vi "三转换ROI对比2.vi"() -> ()   [LabVIEW 2018]
uses:
  <vilib>/vision/NI_Vision_Development_Module.lvlib
panel:
  out "Image 4":T1(plugin-control)
  out "Image 3":T1(plugin-control)
  out "Image 2":T1(plugin-control)
  out "error out":errorcluster
  out "元素":T2 {"Contours"."Type" items=["No Selection", "Point", "Line", "Rectangle", "Oval", "Polygon", "Freehand Region", "Annulus", "Unused2", "Unused3", "Broken Line", "Freehand Line", "Rotated Rectangle"]}
  in  "索引":i32
  out "Image":T1(plugin-control)
  in  "路径":path
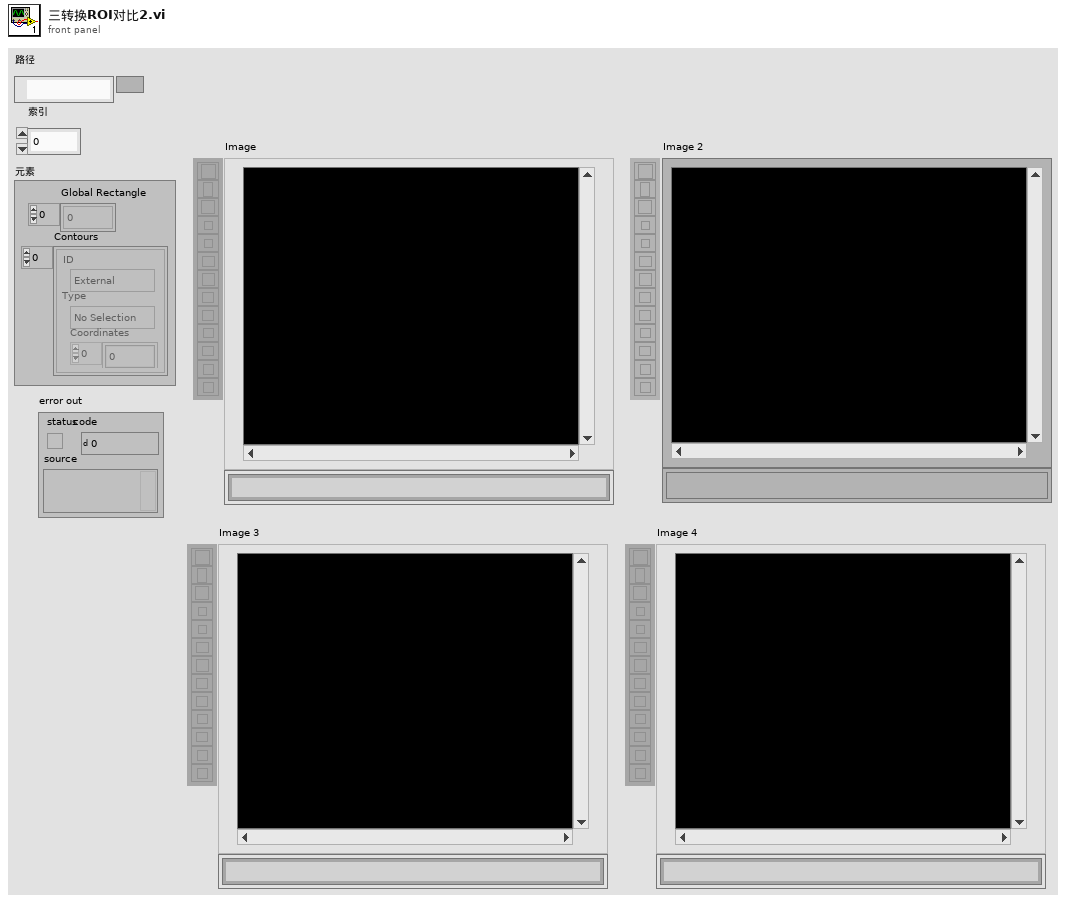
[diagram p1: front panel]
types:
  T1 = typedef "IMAQ Image.ctl" = refnum<image>
  T2 = typedef "ROI Descriptor" = cluster{"Global Rectangle":i32[], "Contours":cluster{"ID":enum32{"External", "Internal"}, "Type":u32, "Coordinates":i32[]}[]}
  T3 = typedef "Image Type" = u32
  T4 = cluster{"ID":enum32{"External", "Internal"}, "Type":u32, "Coordinates":i32[]}[]
  T5 = cluster{"ID":enum32{"External", "Internal"}, "Type":u32, "Coordinates":i32[]}
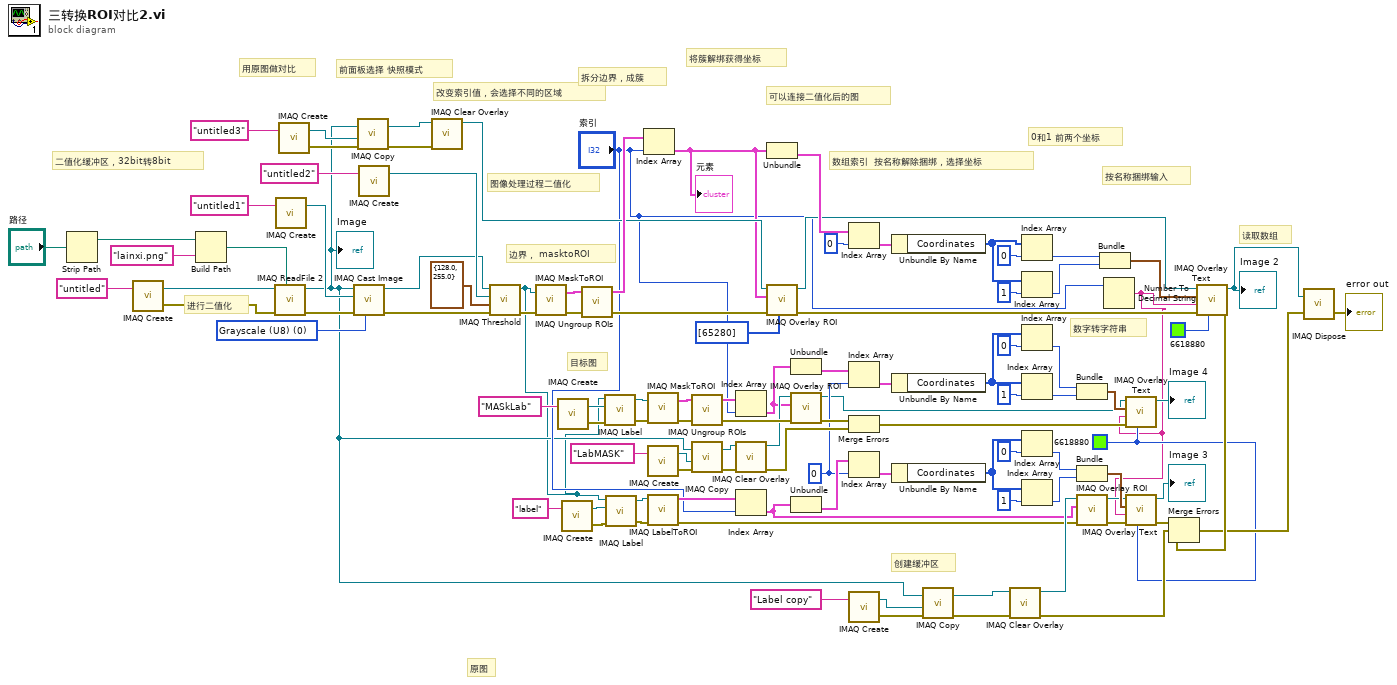
[diagram p0: block diagram]
diagram:
  w6 = u32 6618880 ("Text Color (black)")
  w16 = 0 ("索引")
  w98 = T3 0 items=["Grayscale (U8)", "Grayscale (I16)", "Grayscale (SGL)", "Complex (CSG)", "RGB (U32)", "HSL (U32)", "RGB (U64)", "Grayscale (U16)"] ("Image Type")
  # "目标图"
  # "原图"
  # "创建缓冲区"
  # "改变索引值，会选择不同的区域"
  # "前面板选择 快照模式"
  # "按名称捆绑输入"
  # "读取数组"
  # "0和1 前两个坐标"
  # "数组索引  按名称解除捆绑，选择坐标"
  # "将簇解绑获得坐标"
  # "数字转字符串"
  # "可以连接二值化后的图"
  # "用原图做对比"
  # "拆分边界，成簇"
  # "边界， masktoROI"
  # "图像处理过程二值化"
  # "二值化缓冲区，32bit转8bit"
  # "进行二值化"
  n1 = Strip Path(path="路径") -> (stripped path=w106:path)  [unwired: 1 out]
  n2 = call "IMAQ Create"("Image Name"="untitled") -> ("New Image"=w103:T1, "error out"=w102:errorcluster)  [unwired: 4 in]
  n3 = Build Path(base path=w106, name or relative path="lainxi.png" ("名称或相对路径")) -> (appended path=w104:path)
  n4 = call "IMAQ ReadFile 2"("File Path"=w104, "error in (no error)"=w102, "Image"=w103) -> ("error out"=w97:errorcluster, "Image Out"=w2:T1)  [unwired: 4 in, 3 out]
  "Image" <- w2
  n5 = call "IMAQ Create"("Image Name"="untitled1") -> ("New Image"=w99:T1)  [unwired: 4 in, 1 out]
  n6 = call "IMAQ Create"("Image Name"="untitled3") -> ("New Image"=w85:T1, "error out"=w84:errorcluster)  [unwired: 4 in]
  n7 = call "IMAQ Cast Image"("Image Type"=w98, "error in (no error)"=w97, "Image Dst"=w99, "Image Src"=w2) -> ("error out"=w93:errorcluster, "Image Dst Out"=w95:T1)  [unwired: 6 in]
  n8 = call "IMAQ Copy"("error in (no error)"=w84, "Image Dst"=w85, "Image Src"=w2) -> ("error out"=w82:errorcluster, "Image Dst Out"=w83:T1)  [unwired: 3 in]
  n9 = call "IMAQ Create"("Image Name"="untitled2") -> ("New Image"=w96:T1)  [unwired: 4 in, 1 out]
  n10 = call "IMAQ Clear Overlay"("error in (no error)"=w82, "Image"=w83) -> ("Image Out"=w81:T1)  [unwired: 8 in, 1 out]
  n11 = call "IMAQ Threshold"("error in (no error)"=w93, "Range"=cluster{"Lower value":sgl, "Upper value":sgl} {"Lower value"=128.0, "Upper value"=255.0}, "Image Dst"=w96, "Image Src"=w95) -> ("error out"=w91:errorcluster, "Image Dst Out"=w1:T1)  [unwired: 6 in]
  n12 = call "IMAQ MaskToROI"("Image"=w1, "error in (no error)"=w91) -> ("ROI Descriptor"=w90:T2, "error out"=w89:errorcluster)  [unwired: 5 in, 1 out]
  n13 = call "IMAQ Create"("Image Name"="MASkLab") -> ("New Image"=w25:T1, "error out"=w27:errorcluster)  [unwired: 4 in]
  n14 = call "IMAQ Create"("Image Name"="label") -> ("New Image"=w34:T1, "error out"=w63:errorcluster)  [unwired: 4 in]
  n15 = call "IMAQ Ungroup ROIs"("error in (no error)"=w89, "ROI Descriptor"=w90) -> ("error out"=w87:errorcluster, "ROI Descriptors out"=w88:T2[])  [unwired: 2 in]
  n16 = call "IMAQ Label"("error in (no error)"=w27, "Image Dst"=w25, "Image Src"=w1) -> ("error out"=w28:errorcluster, "Image Dst Out"=w29:T1)  [unwired: 1 in, 1 out]
  n17 = call "IMAQ Label"("error in (no error)"=w63, "Image Dst"=w34, "Image Src"=w1) -> ("error out"=w61:errorcluster, "Image Dst Out"=w62:T1)  [unwired: 1 in, 1 out]
  n18 = Index Array(array=w88, index="索引") -> (element=w80:T2)
  "元素" <- w80
  n19 = call "IMAQ MaskToROI"("Image"=w29, "error in (no error)"=w28) -> ("ROI Descriptor"=w31:T2, "error out"=w30:errorcluster)  [unwired: 5 in, 1 out]
  n20 = call "IMAQ Create"("Image Name"="LabMASK") -> ("New Image"=w3:T1, "error out"=w35:errorcluster)  [unwired: 4 in]
  n21 = call "IMAQ LabelToROI"("error in (no error)"=w61, "Image"=w62) -> ("error out"=w53:errorcluster, "ROIs"=w60:T2[])  [unwired: 6 in, 2 out]
  n22 = call "IMAQ Ungroup ROIs"("error in (no error)"=w30, "ROI Descriptor"=w31) -> ("error out"=w22:errorcluster, "ROI Descriptors out"=w24:T2[])  [unwired: 2 in]
  n23 = call "IMAQ Copy"("error in (no error)"=w35, "Image Dst"=w3, "Image Src"=w2) -> ("error out"=w32:errorcluster, "Image Dst Out"=w33:T1)  [unwired: 3 in]
  n24 = Index Array(array=w24, index="索引") -> (element=w18:T2)
  n25 = call "IMAQ Clear Overlay"("error in (no error)"=w32, "Image"=w33) -> ("error out"=w19:errorcluster, "Image Out"=w21:T1)  [unwired: 8 in]
  n26 = Index Array(array=w60, index="索引") -> (element=w52:T2)
  n27 = Unbundle(w80) -> ("Contours"=w79:T4)  [unwired: 1 out]
  n28 = call "IMAQ Overlay ROI"("Colors (Green)"=u32[] [65280], "error in (no error)"=w87, "ROI Descriptor"=w80, "Image"=w81) -> ("error out"=w70:errorcluster, "Image Out"=w69:T1)  [unwired: 6 in]
  n29 = Unbundle(w18) -> ("Contours"=w17:T4)  [unwired: 1 out]
  n30 = call "IMAQ Overlay ROI"("error in (no error)"=w22, "ROI Descriptor"=w18, "Image"=w21) -> ("error out"=w20:errorcluster, "Image Out"=w8:T1)  [unwired: 7 in]
  n31 = Unbundle(w52) -> ("Contours"=w51:T4)  [unwired: 1 out]
  n32 = Index Array(array=w79, index=0 ("索引")) -> (element=w77:T5)
  n33 = Index Array(array=w17, index=w16) -> (element=w15:T5)
  n34 = Merge Errors(w20, w19) -> (w7:errorcluster)
  n35 = Index Array(array=w51, index=w16) -> (element=w50:T5)
  n36 = call "IMAQ Create"("Image Name"="Label copy") -> ("New Image"=w59:T1, "error out"=w57:errorcluster)  [unwired: 4 in]
  n37 = Unbundle By Name(w77) -> ("Coordinates"=w74:i32[])
  n38 = Unbundle By Name(w15) -> ("Coordinates"=w14:i32[])
  n39 = Unbundle By Name(w50) -> ("Coordinates"=w47:i32[])
  n40 = call "IMAQ Copy"("error in (no error)"=w57, "Image Dst"=w59, "Image Src"=w2) -> ("error out"=w55:errorcluster, "Image Dst Out"=w56:T1)  [unwired: 3 in]
  n41 = call "IMAQ Clear Overlay"("error in (no error)"=w55, "Image"=w56) -> ("error out"=w40:errorcluster, "Image Out"=w54:T1)  [unwired: 8 in]
  n42 = Index Array(array=w74, index=0 ("索引")) -> (element=w73:i32)
  n43 = Index Array(array=w74, index=1 ("索引")) -> (element=w72:i32)
  n44 = Index Array(array=w14, index=0 ("索引")) -> (element=w11:i32)
  n45 = Index Array(array=w14, index=1 ("索引")) -> (element=w10:i32)
  n46 = Index Array(array=w47, index=0 ("索引")) -> (element=w46:i32)
  n47 = Index Array(array=w47, index=1 ("索引")) -> (element=w45:i32)
  n48 = Bundle(w11, w10) -> (w9:cluster{i32, i32})  [unwired: 1 in]
  n49 = Bundle(w46, w45) -> (w44:cluster{i32, i32})  [unwired: 1 in]
  n50 = call "IMAQ Overlay ROI"("error in (no error)"=w53, "ROI Descriptor"=w52, "Image"=w54) -> ("error out"=w42:errorcluster, "Image Out"=w43:T1)  [unwired: 7 in]
  n51 = Bundle(w73, w72) -> (w71:cluster{i32, i32})  [unwired: 1 in]
  n52 = Number To Decimal String(number="索引") -> (decimal integer string=w4:string)  [unwired: 1 in]
  n53 = call "IMAQ Overlay Text"("Text Color (black)"=w6, "error in (no error)"=w7, "String"=w4, "Origin"=w9, "Image"=w8) -> ("Image Out"=→"Image 4":T1)  [unwired: 5 in, 1 out]
  n54 = call "IMAQ Overlay Text"("Text Color (black)"=w6, "error in (no error)"=w42, "String"=w4, "Origin"=w44, "Image"=w43) -> ("error out"=w41:errorcluster, "Image Out"=→"Image 3":T1)  [unwired: 5 in]
  n55 = call "IMAQ Overlay Text"("Text Color (black)"=u32 6618880, "error in (no error)"=w70, "String"=w4, "Origin"=w71, "Image"=w69) -> ("error out"=w39:errorcluster, "Image Out"=w67:T1)  [unwired: 5 in]
  "Image 2" <- w67
  n56 = Merge Errors(w41, w40, w39) -> (w38:errorcluster)
  n57 = call "IMAQ Dispose"("Image"=w67, "error in (no error)"=w38) -> ("error out"=→"error out":errorcluster)  [unwired: 4 in]
